vi "On_pre_tx_flexray_event.vi"(4 "User Parameter":variant, 5 "Event Data":cluster{"AObj":refnum<k24>, "AData":refnum<k24>}, 6 "Control Ref":refnum<k24>, 7 "Event Common Data":T1) -> (1 "Event Data Out":cluster{"AData":refnum<k24>})   [LabVIEW 2018]
uses:
  D:/LabVIEW/TSMaster_FlexRay_Labview/Interop.TSMasterAPI.dll
  Interop.TSMasterAPI.dll
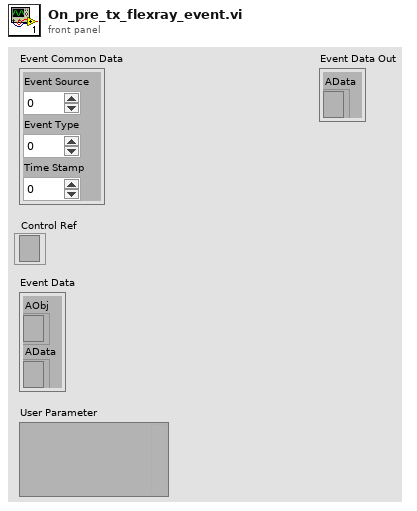
[diagram p1: front panel]
types:
  T1 = cluster{"Event Source":i32, "Event Type":u32, "Time Stamp":u32}
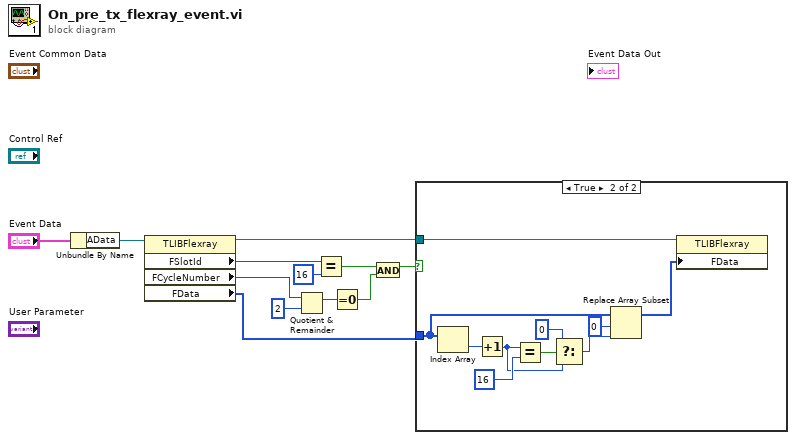
[diagram p0: block diagram]
diagram:
  n1 = Unbundle By Name("Event Data") -> ("AData"=w11:refnum<k24>)
  n2 = property class="TLIBFlexray"(reference=w11) -> (reference out=w7:refnum<k24>, "FSlotId"=w10:u16, "FCycleNumber"=w5:u8, "FData"=w8:u8[])  [unwired: 1 in, 1 out]
  n3 = Quotient & Remainder(x=w5, y=u8 2) -> (x-y*floor(x/y)=w2:u8)  [unwired: 1 out]
  n4 = Equal?(x=w10, y=u16 16) -> (x = y?=w6:bool)
  n5 = Equal To 0?(x=w2) -> (x = 0?=w1:bool)
  n6 = And(x=w6, y=w1) -> (x .and. y?=w3:bool)
  n7 = case shown="True" w3 {
    tunnel: w8 -> [_ w22]
    tunnel: w7 -> [_ w15]
    frame False {
    }
    frame True {
      n8 = Index Array(array=w22) -> (element=w21:u8)  [unwired: 1 in]
      n9 = Increment(x=w21) -> (x+1=w17:u8)
      n10 = Equal?(x=w17, y=u8 16) -> (x = y?=w19:bool)
      n11 = Select(t=u8 0 ("y"), s=w19, f=w17) -> (s? t:f=w16:u8)
      n12 = Replace Array Subset(array=w22, new element=w16, index=0) -> (w14:u8[])
      n13 = property class="TLIBFlexray"(reference=w15, "FData"=w14) -> ()  [unwired: 1 in, 2 out]
    }
  }
